vi "Launch Remote Actor.vi"(6 "Open Actor Core front panel? (F)":bool, 7 "LabVIEW Instance in":refnum<class "LabVIEW Instance.lvclass">, 8 "error in (no error)":errorcluster, 9 "Auto-stop? (T)":bool, 10 "Nested Actor":refnum<class "Actor.lvclass">, 11 "Caller Actor in":refnum<class "Actor.lvclass">) -> (0 "error out":errorcluster, 2 "Nested Actor's Enqueuer":refnum<class "Message Enqueuer.lvclass">, 3 "Caller Actor out":refnum<class "Actor.lvclass">)   [LabVIEW 2014, in "LabVIEW Instance.lvclass"]
uses:
  LabVIEW Instance.lvclass
  <vilib>/ActorFramework/Actor/Actor.lvclass
  <vilib>/ActorFramework/Message Enqueuer/Message Enqueuer.lvclass
  LabVIEW Instance.lvclass/LabVIEW Instance.ctl
  <vilib>/ActorFramework/Upper Proxy Actor/Upper Proxy Actor.lvclass
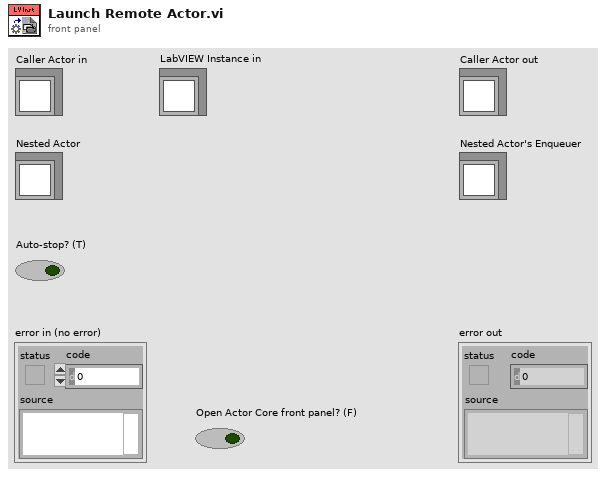
[diagram p1: front panel]
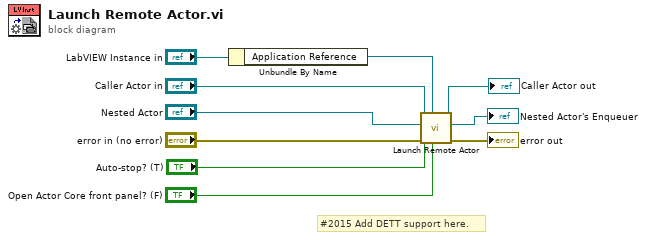
[diagram p0: block diagram]
diagram:
  # "#2015 Add DETT support here."
  n1 = Unbundle By Name("LabVIEW Instance in") -> ("Application Reference"=w1:refnum<vi>)
  n2 = call <vilib>:"Launch Remote Actor.vi"("Open Actor Core front panel? (F)"="Open Actor Core front panel? (F)", "App Refnum"=w1, "error in (no error)"="error in (no error)", "Auto-stop? (T)"="Auto-stop? (T)", "Nested Actor"="Nested Actor", "Caller Actor in"="Caller Actor in") -> ("error out"=→"error out":errorcluster, "Nested Actor's Enqueuer"=→"Nested Actor's Enqueuer":refnum<class "Message Enqueuer.lvclass">, "Caller Actor out"=→"Caller Actor out":refnum<class "Actor.lvclass">)  [unwired: 3 in]
